vi "McP 789A-3 Status V0.49.vi"(8 "error in (no error)":errorcluster) -> (0 "error out":errorcluster, 1 "CurrentPosition":i32, 3 "Velocity (Steps/s)":i32=42372, 11 "PortNumber":i32=1)   [LabVIEW 2024]
doc: "Get Scan velocity and assaign it to the global variable \"McP Scan Velocity\".\nAlso get current stepper reading, etc."
uses:
  Globals and TypeDefs/Global Varibal Control.vi
panel:
  out "X\\r Response":string="XK= 3 I= 25078 V= 49152 \r\r\n"
  in  "IndexM":i32=3
  out "Moving":bool[](array[boolean])=[FALSE, FALSE, FALSE, FALSE, TRUE, TRUE, FALSE, FALSE]
  in  "IndexL":i32=3
  out "Trip Point":i32
  out "Initial Velocity I":i32=801
  out "Ramp Factor K":i32=5
  out "Limits":bool[](array[boolean])=[FALSE, FALSE, FALSE, FALSE, TRUE, TRUE, FALSE, FALSE]
  # "0\n1\n2\n3\n4\n5\n6\n7"
  # "0\n1\n2\n3\n4\n5\n6\n7"
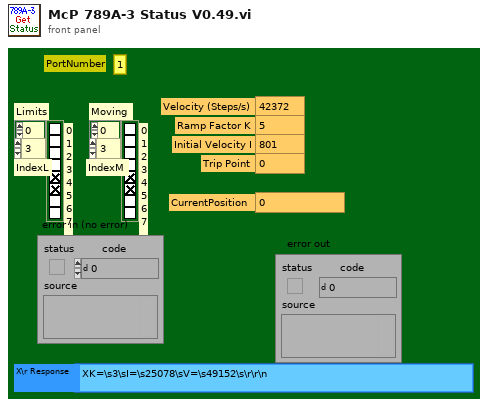
[diagram p1: front panel]
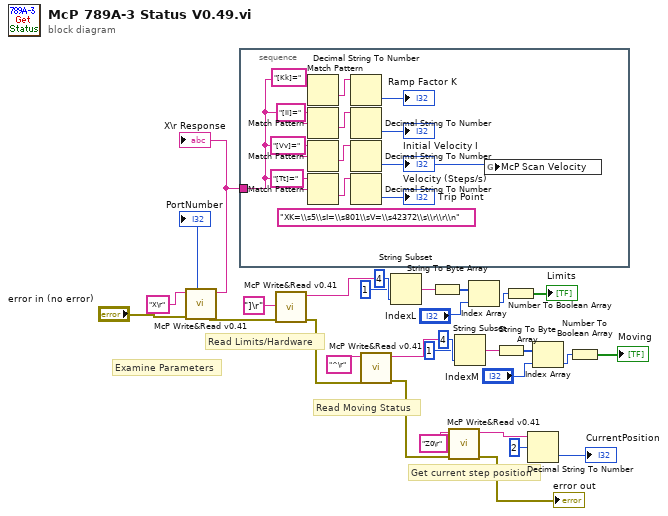
[diagram p0: block diagram]
diagram:
  # "Get current step position"
  # "Examine Parameters"
  # "Read Limits/Hardware"
  # "Read Moving Status"
  n1 = call "McP Write&Read v0.41.vi"("error in (no error)"="error in (no error)", "Write String"="X\r") -> ("error out"=w27:errorcluster, "Read String\nshows:"=w29:string, "PortNumber"=→"PortNumber":i32)  [unwired: 2 in, 2 out]
  "X\\r Response" <- w29
  n2 = stacked-sequence {
    tunnel: w29 -> [w31]
    frame #0 {
      (unwired) "XK=\\s5\\sI=\\s801\\sV=\\s42372\\s\\r\\r\\n"
      n3 = Match Pattern(string=w31, regular expression="[Kk]=") -> (after substring=w36:string)  [unwired: 1 in, 3 out]
      n4 = Match Pattern(string=w31, regular expression="[Ii]=") -> (after substring=w37:string)  [unwired: 1 in, 3 out]
      n5 = Match Pattern(string=w31, regular expression="[Vv]=") -> (after substring=w38:string)  [unwired: 1 in, 3 out]
      n6 = Match Pattern(string=w31, regular expression="[Tt]=") -> (after substring=w39:string)  [unwired: 1 in, 3 out]
      n7 = Decimal String To Number(string=w36) -> (number=→"Ramp Factor K":i32)  [unwired: 2 in, 1 out]
      n8 = Decimal String To Number(string=w37) -> (number=→"Initial Velocity I":i32)  [unwired: 2 in, 1 out]
      n9 = Decimal String To Number(string=w38) -> (number=w41:i32)  [unwired: 2 in, 1 out]
      "Velocity (Steps/s)" <- w41
      n10 = Decimal String To Number(string=w39) -> (number=→"Trip Point":i32)  [unwired: 2 in, 1 out]
      n11 = global write "Global Varibal Control.vi" "McP Scan Velocity"(w41) -> ()
    }
  }
  n12 = call "McP Write&Read v0.41.vi"("error in (no error)"=w27, "Write String"="]\r") -> ("error out"=w16:errorcluster, "Read String\nshows:"=w18:string)  [unwired: 2 in, 3 out]
  n13 = call "McP Write&Read v0.41.vi"("error in (no error)"=w16, "Write String"="^\r") -> ("error out"=w6:errorcluster, "Read String\nshows:"=w8:string)  [unwired: 2 in, 3 out]
  n14 = String Subset(string=w18, offset (0)=1, length (rest)=4) -> (substring=w21:string)
  n15 = String To Byte Array(string=w21) -> (unsigned byte array=w22:u8[])
  n16 = call "McP Write&Read v0.41.vi"("error in (no error)"=w6, "Write String"="Z0\r") -> ("error out"=→"error out":errorcluster, "Read String\nshows:"=w3:string)  [unwired: 2 in, 3 out]
  n17 = String Subset(string=w8, offset (0)=1, length (rest)=4) -> (substring=w11:string)
  n18 = Index Array(array=w22, index="IndexL") -> (element=w23:u8)
  n19 = String To Byte Array(string=w11) -> (unsigned byte array=w12:u8[])
  n20 = Number To Boolean Array(number=w23) -> (Boolean array=→"Limits":bool[])
  n21 = Decimal String To Number(string=w3, offset=2) -> (number=→"CurrentPosition":i32)  [unwired: 1 in, 1 out]
  n22 = Index Array(array=w12, index="IndexM") -> (element=w13:u8)
  n23 = Number To Boolean Array(number=w13) -> (Boolean array=→"Moving":bool[])
